vi "serial write.vi"(8 "error in (no error)":errorcluster, 10 "data":string, 11 "portHandle in":i32) -> (0 "error out":errorcluster, 1 "return value":i32, 3 "portHandle out":i32)   [LabVIEW 2016, in "navX Library.lvlib"]
uses:
  navX Library.lvlib
  libc.so.6
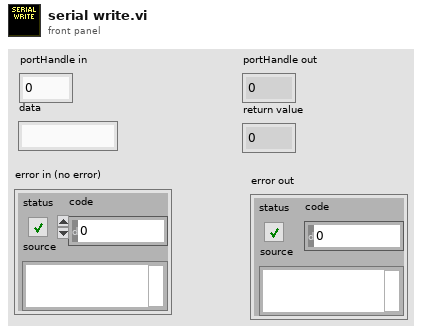
[diagram p1: front panel]
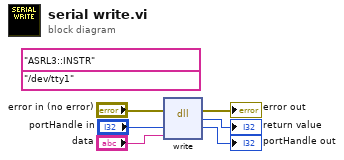
[diagram p0: block diagram]
diagram:
  (unwired) "/dev/tty1"
  (unwired) "ASRL3::INSTR"
  n1 = dll-call lib="libc.so.6" fn="write"(error in="error in (no error)", "portHandle"="portHandle in", "data"="data") -> (error out=→"error out":errorcluster, "return type"=→"return value":i32, "portHandle"=→"portHandle out":i32)  [unwired: 3 in, 1 out]
